vi "Current Loop.vi"(8 "Current Limit":i16, 9 "Gains":T2={"Proportional Gain"=20, "Integral Gain"=10, "Derivative Gain"=0}, 10 "Current Setpoint":i16, 11 "Motor Index":T1) -> ()   [LabVIEW 2011]
doc: "This VI shows an example of how to implement a closed loop position move using the NI 9505. The position loop is implemented using PID. The output of the loop is used as the command for the current loop, which then sets the PWM duty cycle for the motor. This example assumes that an encoder is connected for position and velocity feedback. This example does not implement advanced motion features such as trajectory generation and splining."
uses:
  Controls/Motor Names.ctl
  <vilib>/Platform/TimedLoop/XDataNode/timing_clust.ctl
  <vilib>/Platform/TimedLoop/XDataNode/nitl_modes.ctl
  <vilib>/Platform/TimedLoop/XDataNode/wakeup.ctl
  <vilib>/rvi/Memory/Memory_Emulation/niFpgaMemoryEmulationValidateCache.vi
  <vilib>/rvi/DataTransferAndStorage/Container/Common/niFpgaContainerGetUniqueNameForEmu.vi
  <vilib>/rvi/Memory/Memory_Emulation/nirvimemoryEmulationManagerCache_InsertValue.vi
  <vilib>/Utility/error.llb/Clear Errors.vi
  <vilib>/rvi/Memory/Memory_Emulation/nirvimemoryEmulationManagerCache_GetValue.vi
  <vilib>/rvi/Memory/Memory_Emulation/nirvimemoryEmulationManagerCache_SetValue.vi
  <vilib>/Platform/TimedLoop/XDataNode/XDataNode.xnode
  <vilib>/rvi/DataTransferAndStorage/Container/XNode/niFpgaContainer.xnode
  <vilib>/rvi/Memory/Memory_Emulation/nirvimemoryEmulation.vi
  <vilib>/Platform/TimedLoop/XDataNode/XDNodeRunTimeDep.lvlib
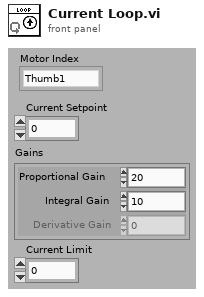
[diagram p1: front panel]
types:
  T1 = typedef "Motor Names.ctl" = enum16{"Thumb1", "Thumb2", "Thumb3", "Middle1", "Middle2", "Middle3", "Redundant", "Index1", "Index2", "Index3"}
  T2 = cluster{"Proportional Gain":i16, "Integral Gain":i16, "Derivative Gain":i16}
  T3 = typedef "XDNodeRunTimeDep.lvlib/timing_clust.ctl" = cluster{"Expected End [f-1]":u64, "Actual End [f-1]":u64, "Finished Late? [f-1]":bool, "Expected End [i-1]":u64, "Actual End [i-1]":u64, "Finished Late? [i-1]":bool, "Expected Start [i]":u64, "Actual Start [i]":u64, "Expected Start [f]":u64, "Actual Start [f]":u64, "Source Name":string, "Structure Name":string, "Period":i64, "Deadline":i64, "Offset":i64, "Start":i64, "Priority":i32, "Timeout":i32, "Mode":T4, "Wakeup Reason":T5, "Error":errorcluster, "Source Type":string, "Secondary Source Type":string, "Global End Time":u64, "Global Start Time":u64, "Frame Duration":u64, "Iteration Duration":u64, "Assigned CPU":i32, "I/O Scan Engine Mode":u32}
  T4 = typedef "XDNodeRunTimeDep.lvlib/nitl_modes.ctl" = enum32{"No Change", "Process missed periods, maintain original phase", "Discard missed periods, maintain original phase", "Process missed periods, ignore original phase", "Discard missed periods, ignore original phase"}
  T5 = typedef "XDNodeRunTimeDep.lvlib/wakeup.ctl" = enum32{"Normal", "Aborted", "Asynchronous wakeup", "Timing source error", "Timed loop error", "Timeout"}
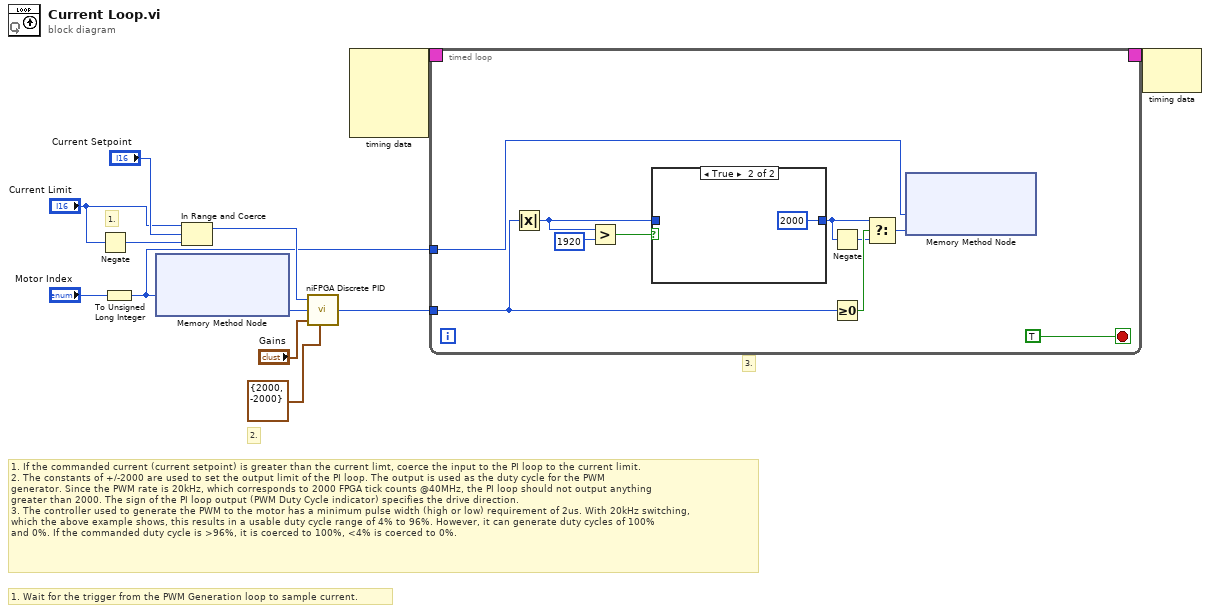
[diagram p0: block diagram]
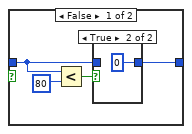
[diagram p2: hidden frame]
diagram:
  # "3."
  # "2."
  # "1."
  # "1. Wait for the trigger from the PWM Generation loop to sample current."
  # "1. If the commanded current (current setpoint) is greater than the current limt, coerce the input to the PI loop to the current limit.\n2. The constants of +/-2000 are used to set the output limit of the PI loop. The output is used as the duty cycle for the PWM\ngenerator. Since the PWM rate is 20kHz, which corresponds to 2000 FPGA tick counts @40MHz, the PI loop should not output anything\ngreater than 2000. The sign of the PI loop output (PWM Duty Cycle indicator) specifies the drive direction.\n3. The controller used to generate the PWM to the motor has a minimum pulse width (high or low) requirement of 2us. With 20kHz switching,\nwhich the above example shows, this results in a usable duty cycle range of 4% to 96%. However, it can generate duty cycles of 100%\nand 0%. If the commanded duty cycle is >96%, it is coerced to 100%, <4% is coerced to 0%."
  n1 = Negate(x="Current Limit") -> (-x=w8:i16)
  n2 = To Unsigned Long Integer(number="Motor Index") -> (unsigned 32bit integer=w3:u32)
  n3 = xnode ("Memory Method Node")("Address"=w3) -> ("Data"=w4:i16)  [unwired: 1 in, 1 out]
  n4 = In Range and Coerce(upper limit="Current Limit", x="Current Setpoint", lower limit=w8) -> (coerced(x)=w7:i16)  [unwired: 1 out]
  n5 = call <vilib>:"niFPGA Discrete PID.vi"("setpoint"=w7, "process variable"=w4, "PID gains (x 2^8)"="Gains", "output range"=cluster{"output high":i16, "output low":i16} {"output high"=2000, "output low"=-2000}) -> ("output"=w9:i16)  [unwired: 1 in, 4 out]
  n6 = node-c288() -> (w12:T3)  [unwired: 4 out]
  n7 = timed-loop {
    timing: w12 -> [_]
    timing-out: [_] -> w11
    tunnel: w9 -> [w16]
    tunnel: w3 -> [w14]
    stop <- TRUE stop-if-true
    n8 = Absolute Value(x=w16) -> (abs(x)=w17:i16)
    n9 = Greater?(x=w17, y=i16 1920 ("upper limit")) -> (0:w19:bool)
    n10 = case shown="True" w19 {
      tunnel: [w25 i16 2000 ("upper limit")] -> w18
      tunnel: w17 -> [w23 _]
      frame False {
        n11 = Less?(x=w23, y=i16 80 ("lower limit")) -> (x < y?=w24:bool)
        n12 = case shown="True" w24 {
          tunnel: [w27 i16 0 ("upper limit")] -> w25
          tunnel: w23 -> [w27 _]
          frame False {
          }
          frame True {
          }
        }
      }
      frame True {
      }
    }
    n13 = Negate(x=w18) -> (-x=w21:i16)
    n14 = Greater Or Equal To 0?(x=w16) -> (x >= 0?=w22:bool)
    n15 = Select(t=w18, s=w22, f=w21) -> (s? t:f=w13:i16)
    n16 = xnode ("Memory Method Node")("Address"=w14, "Data"=w13) -> ()  [unwired: 1 in, 1 out]
  }
  n17 = node-c288(w11) -> ()  [unwired: 1 out]
